vi "Get All Names from Database.vi"(8 "error in (no error)":errorcluster, 11 "database in (:memory:)":refnum<k21>=":memory:") -> (0 "error out":errorcluster, 2 "Cluster":T1, 3 "XNET Database":refnum<k21>)   [LabVIEW 2015]
uses:
  controls/dbc-content-data.ctl
  <resource>/objmgr/xnet.rc
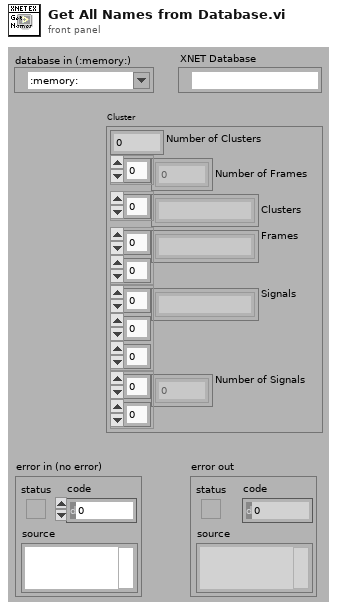
[diagram p1: front panel]
types:
  T1 = typedef "dbc-content-data.ctl" = cluster{"Number of Clusters":i32, "Number of Frames ":i32[], "Clusters":string[], "Frames":string[][], "Signals":string[][][], "Number of Signals":i32[][]}
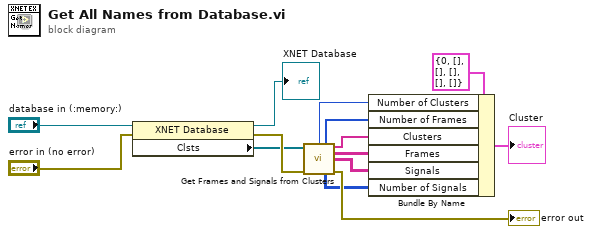
[diagram p0: block diagram]
diagram:
  n1 = property class="XNET Database"(reference="database in (:memory:)", error in="error in (no error)") -> (reference out=→"XNET Database":refnum<k21>, error out=w14:errorcluster, "Clsts"=w8:refnum<k21>[])
  n2 = call "Get Frames and Signals from Clusters.vi"("XNET Clusters"=w8, "error in"=w14) -> ("Number of Clusters"=w6:i32, "Number of Frames"=w5:i32[], "Cluster Names"=w3:string[], "Frame Names"=w2:string[][], "Signal Names"=w1:string[][][], "Number of Signals"=w4:i32[][], "error out"=→"error out":errorcluster)  [unwired: 2 in, 5 out]
  n3 = Bundle By Name(cluster=T1 {"Number of Clusters"=0, "Number of Frames "=[], "Clusters"=[], "Frames"=[], "Signals"=[], "Number of Signals"=[]} ("Cluster"), "Number of Clusters"=w6, "Number of Frames"=w5, "Clusters"=w3, "Frames"=w2, "Signals"=w1, "Number of Signals"=w4) -> (→"Cluster":T1)
